vi "Initialize SPI Internal References.vi"(8 "error in":errorcluster, 9 "SPI Engine Source":refnum<k21>, 10 "SPI PHY Settings":T5={"Divide Value"=0, "Transfer Length (bits)"=1, "CS Asserted Polarity"=FALSE, "Clock Polarity (CPOL)"=FALSE, "Clock Phase (CPHA)"=FALSE, "Lengthen MISO Setup"=FALSE, "Direction Change Bit"=0, "MOSI Starts as Output"=FALSE, "Tristatable MOSI"=FALSE} {"Direction Change Bit" max=64 step=1; "Transfer Length (bits)" min=1 max=64 step=1}, 11 "SPI Signal Settings":T2={"SCLK"={"Signal"="sbRIO-9651 Socket\\PMOD1_Pin4_out", "Signal_Enable"="sbRIO-9651 Socket\\PMOD1_Pin4_enable", "Output?"=FALSE}, "Signal Settings"={"MISO"="sbRIO-9651 Socket\\PMOD1_Pin3_in", "Signal_Enable"="sbRIO-9651 Socket\\PMOD1_Pin4_enable", "Output?"=FALSE}, "MOSI"={"Signal"="sbRIO-9651 Socket\\PMOD1_Pin4_out", "Signal_Enable"="sbRIO-9651 Socket\\PMOD1_Pin4_enable", "Output?"=FALSE}, "CS0"={"Signal"="sbRIO-9651 Socket\\PMOD1_Pin4_out", "Signal_Enable"="sbRIO-9651 Socket\\PMOD1_Pin4_enable", "Output?"=FALSE}, "CS1"={"Signal"="sbRIO-9651 Socket\\PMOD1_Pin4_out", "Signal_Enable"="sbRIO-9651 Socket\\PMOD1_Pin4_enable", "Output?"=FALSE}, "CS2"={"Signal"="sbRIO-9651 Socket\\PMOD1_Pin4_out", "Signal_Enable"="sbRIO-9651 Socket\\PMOD1_Pin4_enable", "Output?"=FALSE}, "CS3"={"Signal"="sbRIO-9651 Socket\\PMOD1_Pin4_out", "Signal_Enable"="sbRIO-9651 Socket\\PMOD1_Pin4_enable", "Output?"=FALSE}, "CS4"={"Signal"="sbRIO-9651 Socket\\PMOD1_Pin4_out", "Signal_Enable"="sbRIO-9651 Socket\\PMOD1_Pin4_enable", "Output?"=FALSE}, "CS5"={"Signal"="sbRIO-9651 Socket\\PMOD1_Pin4_out", "Signal_Enable"="sbRIO-9651 Socket\\PMOD1_Pin4_enable", "Output?"=FALSE}}) -> (0 "error out":errorcluster, 3 "SPI Engine Reference":T1={"SPI Signal Settings"={"SCLK"={"Signal"="sbRIO-9651 Socket\\PMOD1_Pin4_out", "Signal_Enable"="sbRIO-9651 Socket\\PMOD1_Pin4_enable", "Output?"=FALSE}, "Signal Settings"={"MISO"="sbRIO-9651 Socket\\PMOD1_Pin3_in", "Signal_Enable"="sbRIO-9651 Socket\\PMOD1_Pin4_enable", "Output?"=FALSE}, "MOSI"={"Signal"="sbRIO-9651 Socket\\PMOD1_Pin4_out", "Signal_Enable"="sbRIO-9651 Socket\\PMOD1_Pin4_enable", "Output?"=FALSE}, "CS0"={"Signal"="sbRIO-9651 Socket\\PMOD1_Pin4_out", "Signal_Enable"="sbRIO-9651 Socket\\PMOD1_Pin4_enable", "Output?"=FALSE}, "CS1"={"Signal"="sbRIO-9651 Socket\\PMOD1_Pin4_out", "Signal_Enable"="sbRIO-9651 Socket\\PMOD1_Pin4_enable", "Output?"=FALSE}, "CS2"={"Signal"="sbRIO-9651 Socket\\PMOD1_Pin4_out", "Signal_Enable"="sbRIO-9651 Socket\\PMOD1_Pin4_enable", "Output?"=FALSE}, "CS3"={"Signal"="sbRIO-9651 Socket\\PMOD1_Pin4_out", "Signal_Enable"="sbRIO-9651 Socket\\PMOD1_Pin4_enable", "Output?"=FALSE}, "CS4"={"Signal"="sbRIO-9651 Socket\\PMOD1_Pin4_out", "Signal_Enable"="sbRIO-9651 Socket\\PMOD1_Pin4_enable", "Output?"=FALSE}, "CS5"={"Signal"="sbRIO-9651 Socket\\PMOD1_Pin4_out", "Signal_Enable"="sbRIO-9651 Socket\\PMOD1_Pin4_enable", "Output?"=FALSE}}, "SPI Internal Signals"={"DLU To SPI Engine Data FIFO"="DLU To SPI Engine Data", "SPI Engine to DLU Data FIFO"="SPI Engine to DLU Data", "Data to SPI Engine (Cache) Register"="Data to SPI Engine (Cache)", "SPI PHY Settings to SPI Engine (Cahche) Register"="SPI PHY Settings to SPI Engine (Cache)"}, "SPI PHY Settings"={"Divide Value"=0, "Transfer Length (bits)"=0, "CS Asserted Polarity"=FALSE, "Clock Polarity (CPOL)"=FALSE, "Clock Phase (CPHA)"=FALSE, "Lengthen MISO Setup"=FALSE, "Direction Change Bit"=0, "MOSI Starts as Output"=FALSE, "Tristatable MOSI"=FALSE}, "SPI Engine Source"="120MHz"} {"SPI PHY Settings"."Direction Change Bit" max=64 step=1; "SPI PHY Settings"."Transfer Length (bits)" min=1 max=64 step=1})   [LabVIEW 2014]
uses:
  Controls/SPI Settings.ctl
  Controls/Signal Properties.ctl
  <userlib>/_NI SPI IP/FPGA/Controllers/Public/Transfer Settings.ctl
  Controls/All SPI Settings.ctl
  Controls/Internal Data (SPI API).ctl
  <vilib>/rvi/DataTransferAndStorage/Container/Common/niFpgaContainerGetUniqueNameForEmu.vi
  <vilib>/rvi/DataTransferAndStorage/Container/Common/niFpgaContainerSetEmuInfo.vi
  <vilib>/rvi/eio/common/nirviEmuReportErrorAndStop.vi
  <vilib>/rvi/LocalResourceManager/LocalResourceManager.xnode
  <userlib>/_NI SPI IP/FPGA/Controllers/NI SPI IP FPGA.lvlib
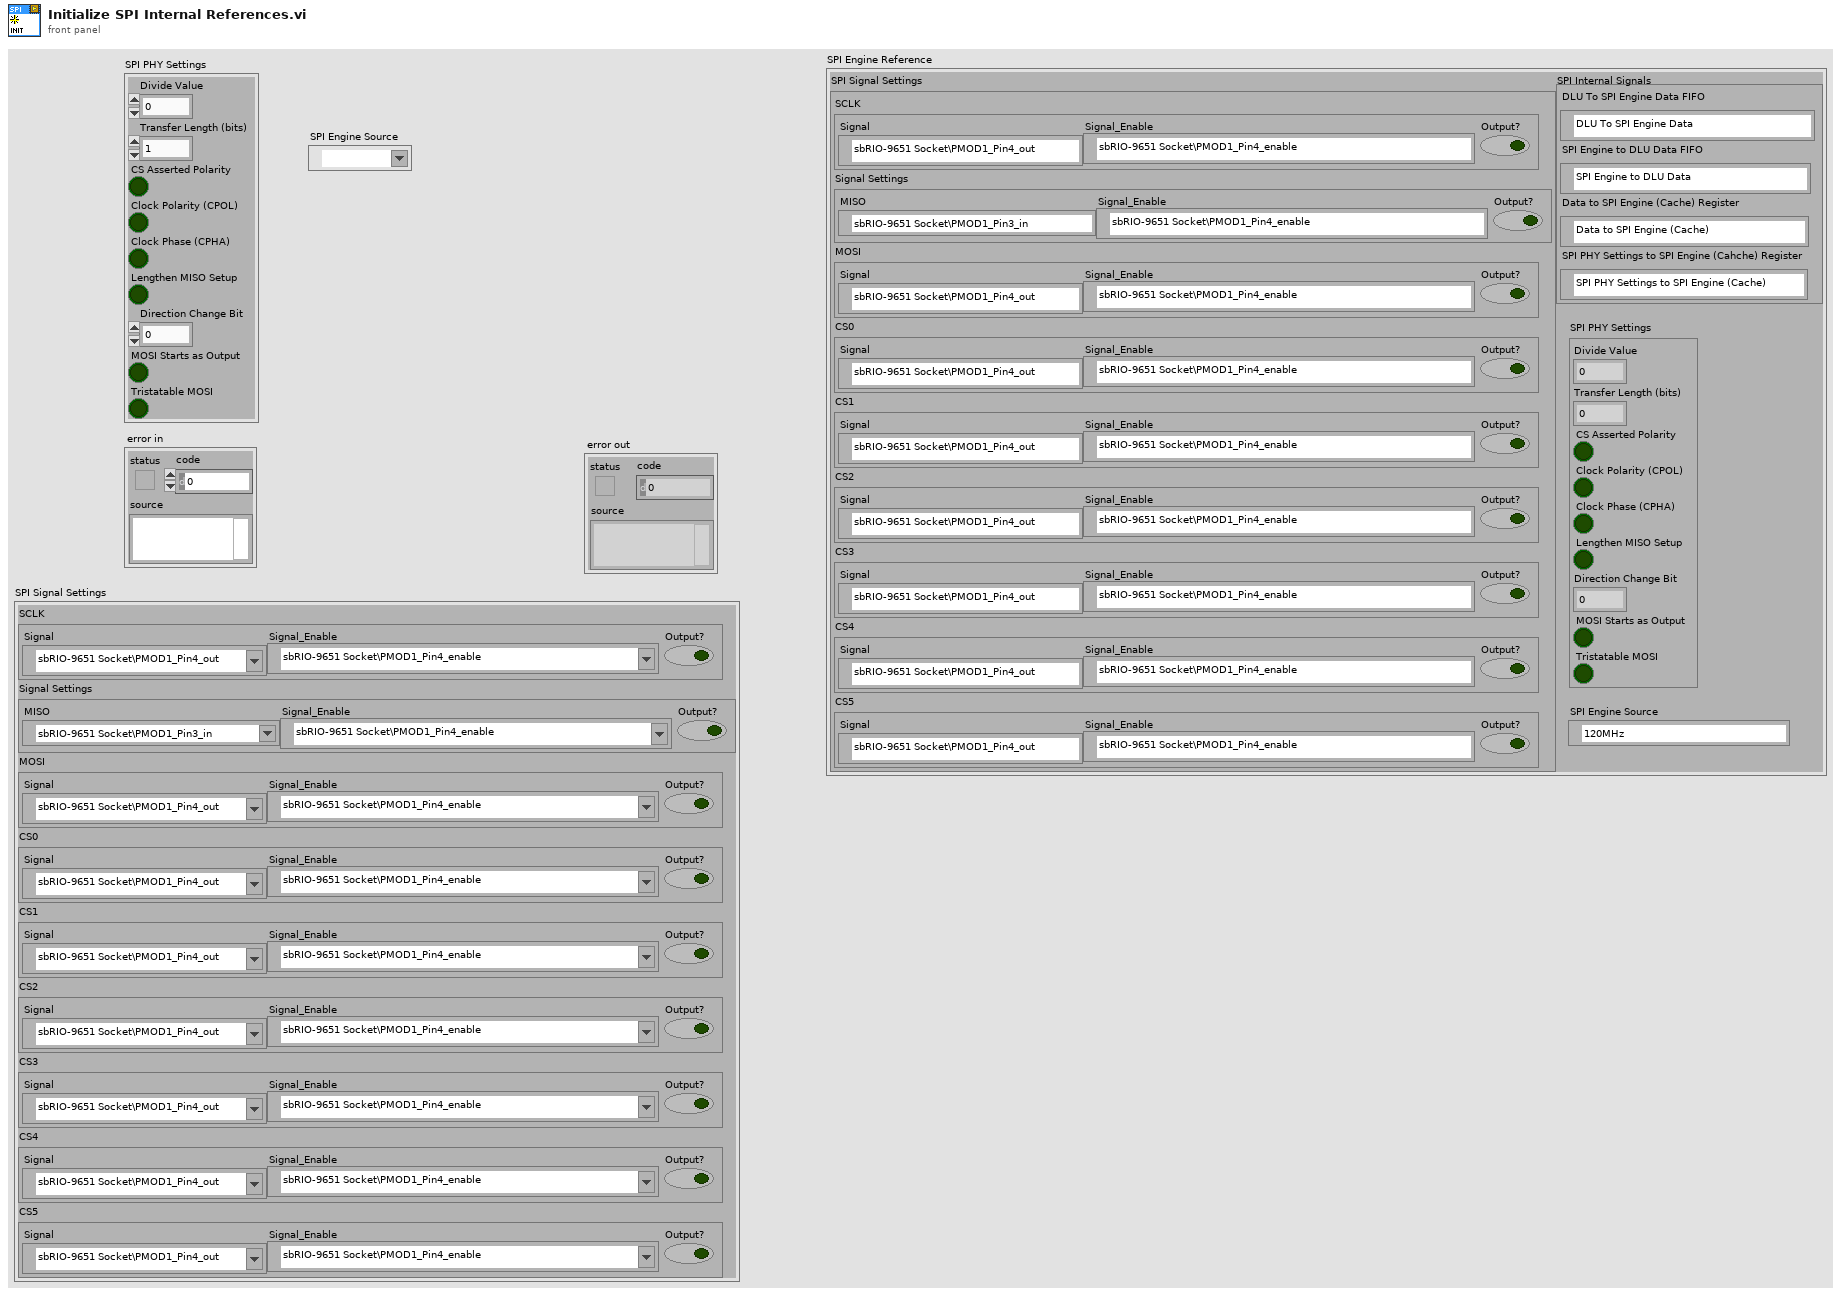
[diagram p1: front panel]
types:
  T1 = typedef "All SPI Settings.ctl" = cluster{"SPI Signal Settings":T2, "SPI Internal Signals":T4, "SPI PHY Settings":T5, "SPI Engine Source":refnum<k21>}
  T2 = typedef "SPI Settings.ctl" = cluster{"SCLK":T3, "Signal Settings":cluster{"MISO":refnum<k21>, "Signal_Enable":refnum<k21>, "Output?":bool}, "MOSI":T3, "CS0":T3, "CS1":T3, "CS2":T3, "CS3":T3, "CS4":T3, "CS5":T3}
  T3 = typedef "Signal Properties.ctl" = cluster{"Signal":refnum<k21>, "Signal_Enable":refnum<k21>, "Output?":bool}
  T4 = typedef "Internal Data (SPI API).ctl" = cluster{"DLU To SPI Engine Data FIFO":refnum<k21>, "SPI Engine to DLU Data FIFO":refnum<k21>, "Data to SPI Engine (Cache) Register":refnum<k21>, "SPI PHY Settings to SPI Engine (Cahche) Register":refnum<k21>}
  T5 = typedef "NI SPI IP FPGA.lvlib/Transfer Settings.ctl" = cluster{"Divide Value":u8, "Transfer Length (bits)":u8, "CS Asserted Polarity":bool, "Clock Polarity (CPOL)":bool, "Clock Phase (CPHA)":bool, "Lengthen MISO Setup":bool, "Direction Change Bit":u8, "MOSI Starts as Output":bool, "Tristatable MOSI":bool}
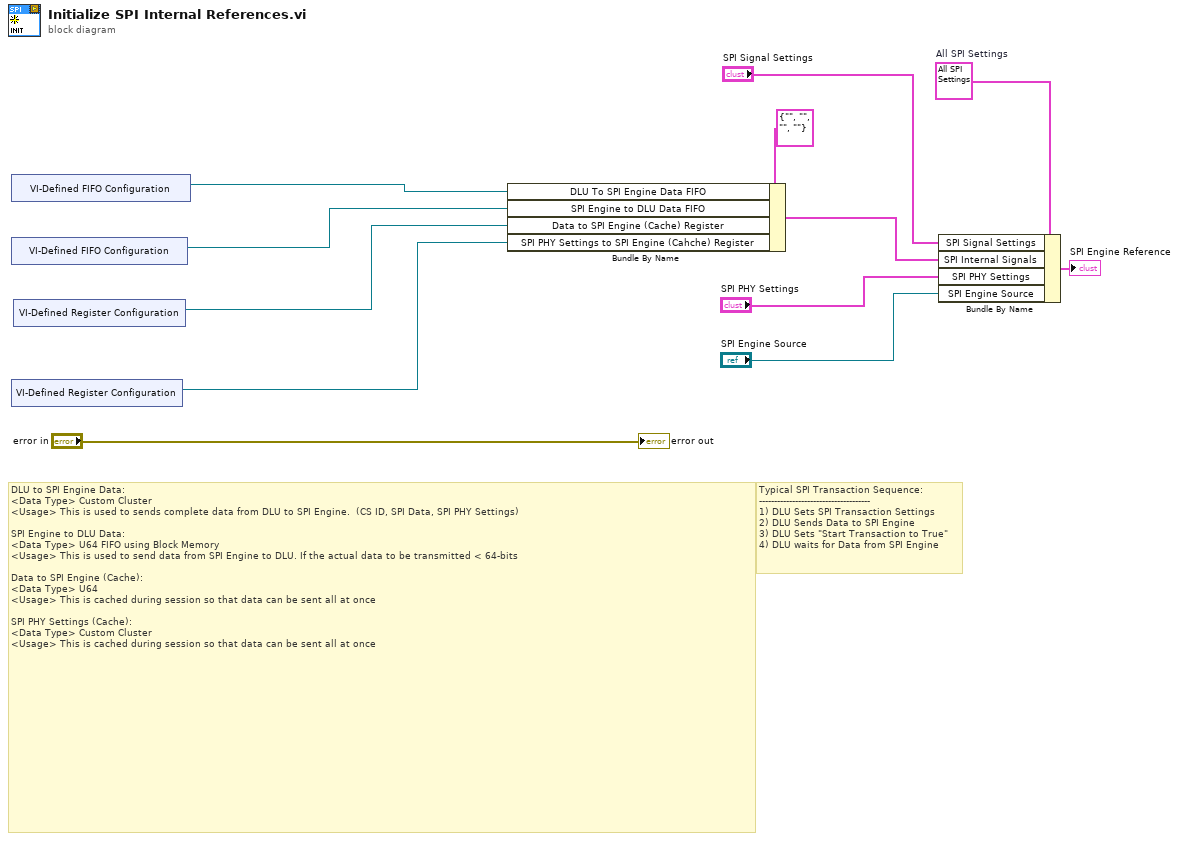
[diagram p0: block diagram]
diagram:
  w6 = T1 {"SPI Signal Settings"={"SCLK"={"Signal"="sbRIO-9651 Socket\\PMOD1_Pin4_out", "Signal_Enable"="sbRIO-9651 Socket\\PMOD1_Pin4_enable", "Output?"=FALSE}, "Signal Settings"={"MISO"="sbRIO-9651 Socket\\PMOD1_Pin3_in", "Signal_Enable"="sbRIO-9651 Socket\\PMOD1_Pin4_enable", "Output?"=FALSE}, "MOSI"={"Signal"="sbRIO-9651 Socket\\PMOD1_Pin4_out", "Signal_Enable"="sbRIO-9651 Socket\\PMOD1_Pin4_enable", "Output?"=FALSE}, "CS0"={"Signal"="sbRIO-9651 Socket\\PMOD1_Pin4_out", "Signal_Enable"="sbRIO-9651 Socket\\PMOD1_Pin4_enable", "Output?"=FALSE}, "CS1"={"Signal"="sbRIO-9651 Socket\\PMOD1_Pin4_out", "Signal_Enable"="sbRIO-9651 Socket\\PMOD1_Pin4_enable", "Output?"=FALSE}, "CS2"={"Signal"="sbRIO-9651 Socket\\PMOD1_Pin4_out", "Signal_Enable"="sbRIO-9651 Socket\\PMOD1_Pin4_enable", "Output?"=FALSE}, "CS3"={"Signal"="sbRIO-9651 Socket\\PMOD1_Pin4_out", "Signal_Enable"="sbRIO-9651 Socket\\PMOD1_Pin4_enable", "Output?"=FALSE}, "CS4"={"Signal"="sbRIO-9651 Socket\\PMOD1_Pin4_out", "Signal_Enable"="sbRIO-9651 Socket\\PMOD1_Pin4_enable", "Output?"=FALSE}, "CS5"={"Signal"="sbRIO-9651 Socket\\PMOD1_Pin4_out", "Signal_Enable"="sbRIO-9651 Socket\\PMOD1_Pin4_enable", "Output?"=FALSE}}, "SPI Internal Signals"={"DLU To SPI Engine Data FIFO"="DLU To SPI Engine Data", "SPI Engine to DLU Data FIFO"="SPI Engine to DLU Data", "Data to SPI Engine (Cache) Register"="Data to SPI Engine (Cache)", "SPI PHY Settings to SPI Engine (Cahche) Register"="SPI PHY Settings to SPI Engine (Cache)"}, "SPI PHY Settings"={"Divide Value"=0, "Transfer Length (bits)"=0, "CS Asserted Polarity"=FALSE, "Clock Polarity (CPOL)"=FALSE, "Clock Phase (CPHA)"=FALSE, "Lengthen MISO Setup"=FALSE, "Direction Change Bit"=0, "MOSI Starts as Output"=FALSE, "Tristatable MOSI"=FALSE}, "SPI Engine Source"="120MHz"}  # All SPI Settings
  # "Typical SPI Transaction Sequence:\n-------------------------------------\n1) DLU Sets SPI Transaction Settings\n2) DLU Sends Data to SPI Engine \n3) DLU Sets \"Start Transaction to True\"\n4) DLU waits for Data from SPI Engine"
  # "DLU to SPI Engine Data: \n<Data Type> Custom Cluster\n<Usage> This is used to sends complete data from DLU to SPI Engine.  (CS ID, SPI Data, SPI PHY Settings)\n\nSPI Engine to DLU Data: \n<Data Type> U64 FIFO using Block Memory\n<Usage> This is used to send data from SPI Engine to DLU. If the actual data to be transmitted < 64-bits\n\nData to SPI Engine (Cache):\n<Data Type> U64\n<Usage> This is cached during session so that data can be sent all at once\n\nSPI PHY Settings (Cache):\n<Data Type> Custom Cluster\n<Usage> This is cached during session so that data can be sent all at once"
  n1 = xnode "VI-Defined FIFO Configuration"() -> ("FIFO Out"=w10:refnum<k21>)
  n2 = xnode "VI-Defined FIFO Configuration"() -> ("FIFO Out"=w9:refnum<k21>)
  n3 = xnode ("VI-Defined Register Configuration")() -> ("Register Out"=w7:refnum<k21>)
  n4 = xnode ("VI-Defined Register Configuration")() -> ("Register Out"=w8:refnum<k21>)
  n5 = Bundle By Name(cluster=T4 {"DLU To SPI Engine Data FIFO"="", "SPI Engine to DLU Data FIFO"="", "Data to SPI Engine (Cache) Register"="", "SPI PHY Settings to SPI Engine (Cahche) Register"=""} ("Private Data"), "DLU To SPI Engine Data FIFO"=w10, "SPI Engine to DLU Data FIFO"=w9, "Data to SPI Engine (Cache) Register"=w8, "SPI PHY Settings to SPI Engine (Cahche) Register"=w7) -> (w5:T4)
  n6 = Bundle By Name(cluster=w6, "SPI Signal Settings"="SPI Signal Settings", "SPI Internal Signals"=w5, "SPI PHY Settings"="SPI PHY Settings", "SPI Engine Source"="SPI Engine Source") -> (→"SPI Engine Reference":T1)
  "error out" <- "error in"
